vi "PDF Protokoll EPA1065_InterferenceVerification.vi"(8 "error in (no error)":errorcluster caption="Fehler (Eingang, kein Fehler)") -> (0 "error out":errorcluster caption="Fehler (Ausgang)")   [LabVIEW 2020, in "EPA 1065.lvlib" / "Interference verificaton 1065-375.lvlib"]
uses:
  Interference verificaton 1065-375.lvlib
  Visualisierungs Elemente/String - Ausgabefeld.ctl
  ResultTable.ctl
  Sprachverwaltung/FGV Aktion Tabelle zerlegen.ctl
  <vilib>/Utility/miscctls.llb/LVRowAndColumnTypeDef.ctl
  Aktion FGV Interference.ctl
  Seiten/FT-IR/FGV FT-IR Aktionen.ctl
  Aktion Index uebersetzten.ctl
  Seiten/System Einstellungen V2/Aktioen FGV System Konstanten.ctl
  <vilib>/Utility/miscctls.llb/LVPrintingMarginsTypeDef.ctl
  Allgemein/allgemeine Sub-VIs.lvlib
  Seiten/FT-IR/Span/Spanfaktor.lvlib
  Seiten/FT-IR/FT-IR.lvlib
  Sprachverwaltung/Sprachverwaltung.lvlib
  Seiten/System Einstellungen V2/System Einstellungen V2.lvlib
panel:
  out "[ppm]":sgl=1.0 caption="Limit:" min=0 format="%#.6g"
  out "[ppm]":sgl=120.0 caption="Interference:" min=0 format="%#.6g"
  out "LIN Ausgabetabelle":T1
  out "Komponente:":T2 caption="ppm"
  out "Tabelle 3":string[][](table)
  out "Tabelle":string[][](table)
  # "Interference Verification - EPA § 1065.375"
  # "Result"
  # "Analysis"
  # "Component:"
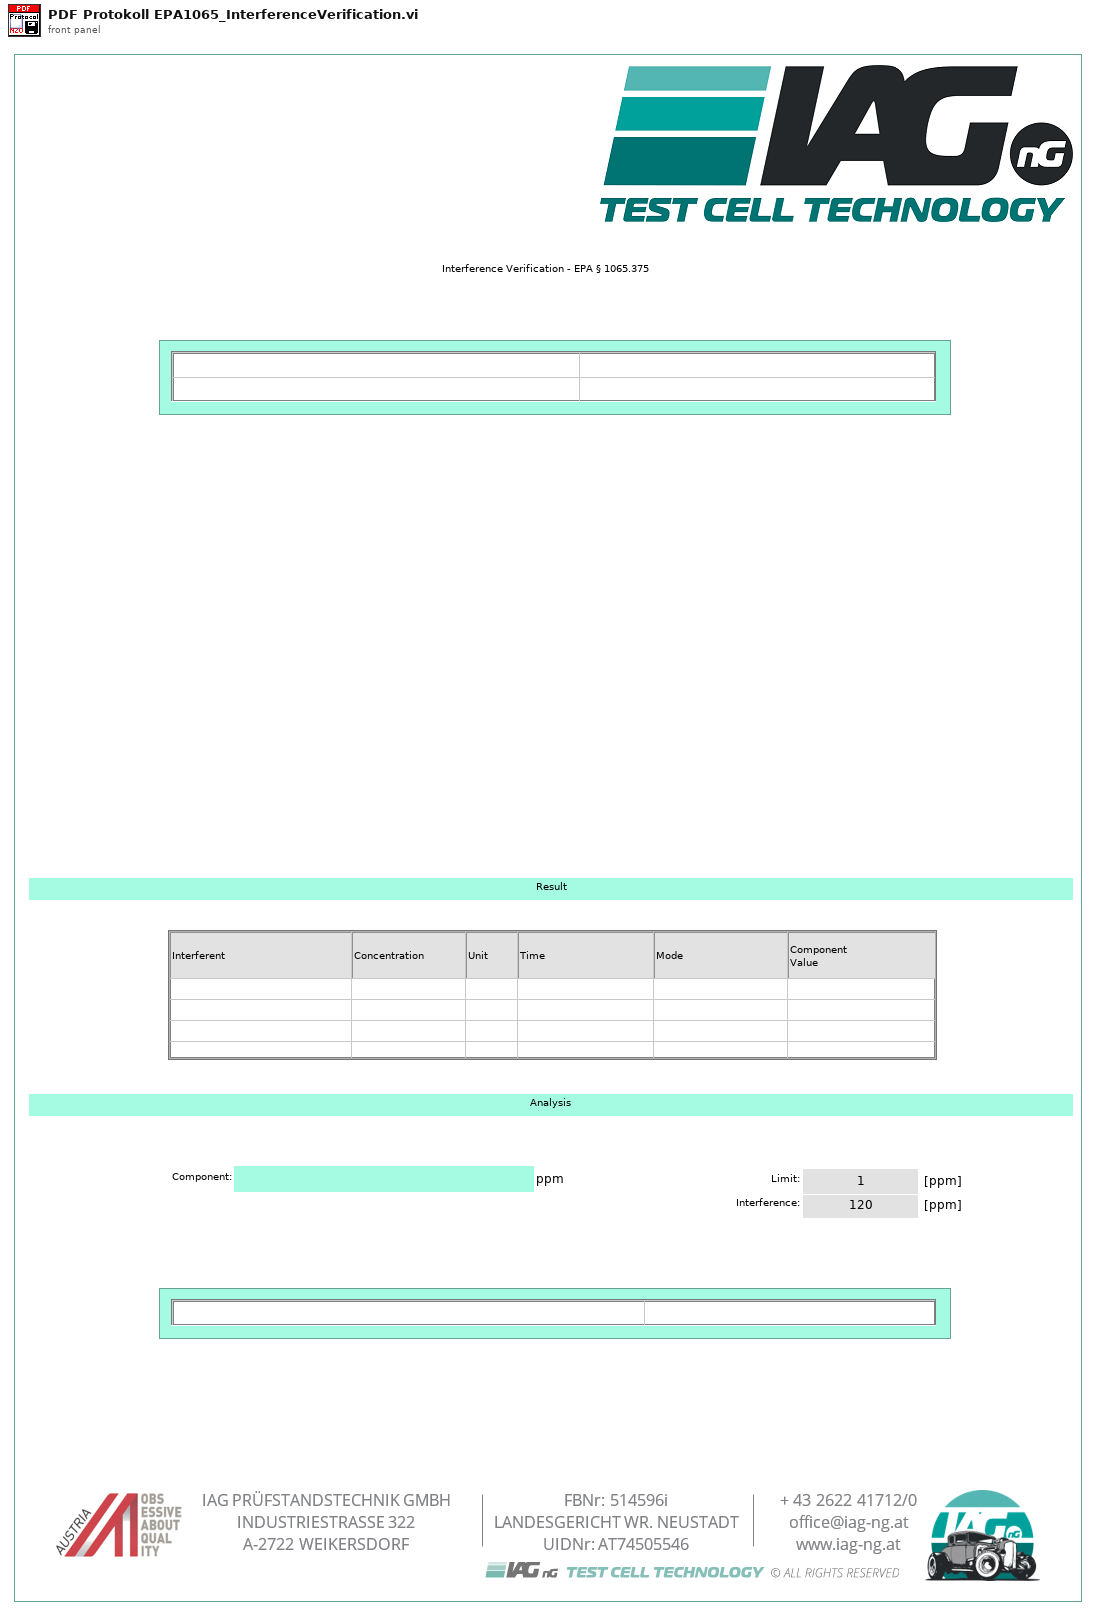
[diagram p1: front panel]
types:
  T1 = typedef "EPA 1065.lvlib/Interference verificaton 1065-375.lvlib/ResultTable.ctl" = string[][]
  T2 = typedef "String - Ausgabefeld.ctl" = string
  T3 = typedef "Sprachverwaltung.lvlib/FGV Aktion Tabelle zerlegen.ctl" = enum16{"laden", "vereinzeln", "speichern"}
  T4 = typedef "System Einstellungen V2.lvlib/Aktioen FGV System Konstanten.ctl" = enum16{"lesen", "laden", "speichern", "Sprache"}
  T5 = typedef "EPA 1065.lvlib/Interference verificaton 1065-375.lvlib/Aktion Index uebersetzten.ctl" = enum16{"lesen", "schreiben", "auswerten"}
  T6 = typedef "FT-IR.lvlib/FGV FT-IR Aktionen.ctl" = enum16{"lesen", "NOG setzen", "NOS setzen", "Initialisieren", "speichern", "ALLES setzen", "FT-IR Spektrum loggen", "Komm Stoppen", "Spektrum LogKonfig"}
  T7 = typedef "EPA 1065.lvlib/Interference verificaton 1065-375.lvlib/Aktion FGV Interference.ctl" = enum16{"Lesen", "TestKonfig", "TestSetting", "Einheiten", "Ergebnis", "Laden", "Tabelle", "Speichern", "löschen"}
  T8 = typedef "LVRowAndColumnTypeDef.ctl" = cluster{"Row":i32, "Column":i32}
  T9 = typedef "LVPrintingMarginsTypeDef.ctl" = cluster{"Top":sgl, "Left":sgl, "Bottom":sgl, "Right":sgl, "Measurement System":enum8{"Inches", "cm"}}
  T10 = enum32{"Portrait", "Landscape", "Rotated Portrait", "Rotated Landscape"}
  T11 = typedef "EPA 1065.lvlib/Interference verificaton 1065-375.lvlib/TestSetting.ctl" = cluster{"Bearbeiter:":string, "Pfad:":path, "Textname:":string, "Analysator":T12}
  T12 = typedef "System Einstellungen V2.lvlib/Analysatoren.ctl" = string
  T13 = typedef "EPA 1065.lvlib/Interference verificaton 1065-375.lvlib/TestKonfig.ctl" = cluster{"Komponente:":u16, "Modus":T14, "CG Aufschaltzeit:":dbl, "Interferent 1:":u16, "Interferent 2:":u16, "Interferent 3:":u16, "Gasflaschen Nr.:":string, "Gasflaschen Nr.: 2":string, "Gasflaschen Nr.: 3":string, "Inter 1 aktiv":bool, "Inter 2 aktiv":bool, "Inter 3 aktiv":bool, "Accuracy":string, "Accuracy 2":string, "Accuracy 3":string, "Konzentration 1:":dbl, "Konzentration 2:":dbl, "Konzentration 3:":dbl}
  T14 = typedef "EPA 1065.lvlib/Interference verificaton 1065-375.lvlib/Modus.ctl" = u16
  T15 = typedef "EPA 1065.lvlib/Interference verificaton 1065-375.lvlib/Komponenten.ctl" = cluster{"Komponente":T2, "Komponente Index":i32, "Komponente 2":T2, "Komponente Index 2":i32, "Komponente 3":T2, "Komponente Index 3":i32, "Interferent 1":T2, "Interferent Index":i32, "Interferent 2":T2, "Interferent 2 Index":i32, "Interferent 3":T2, "Interferent 3 Index":i32, "Interferent 4":T2, "Interferent 4 Index":i32}
  T16 = cluster{"Modell":string, "ProjektNummer":string, "Software Version":string, "Seriennummer":string}
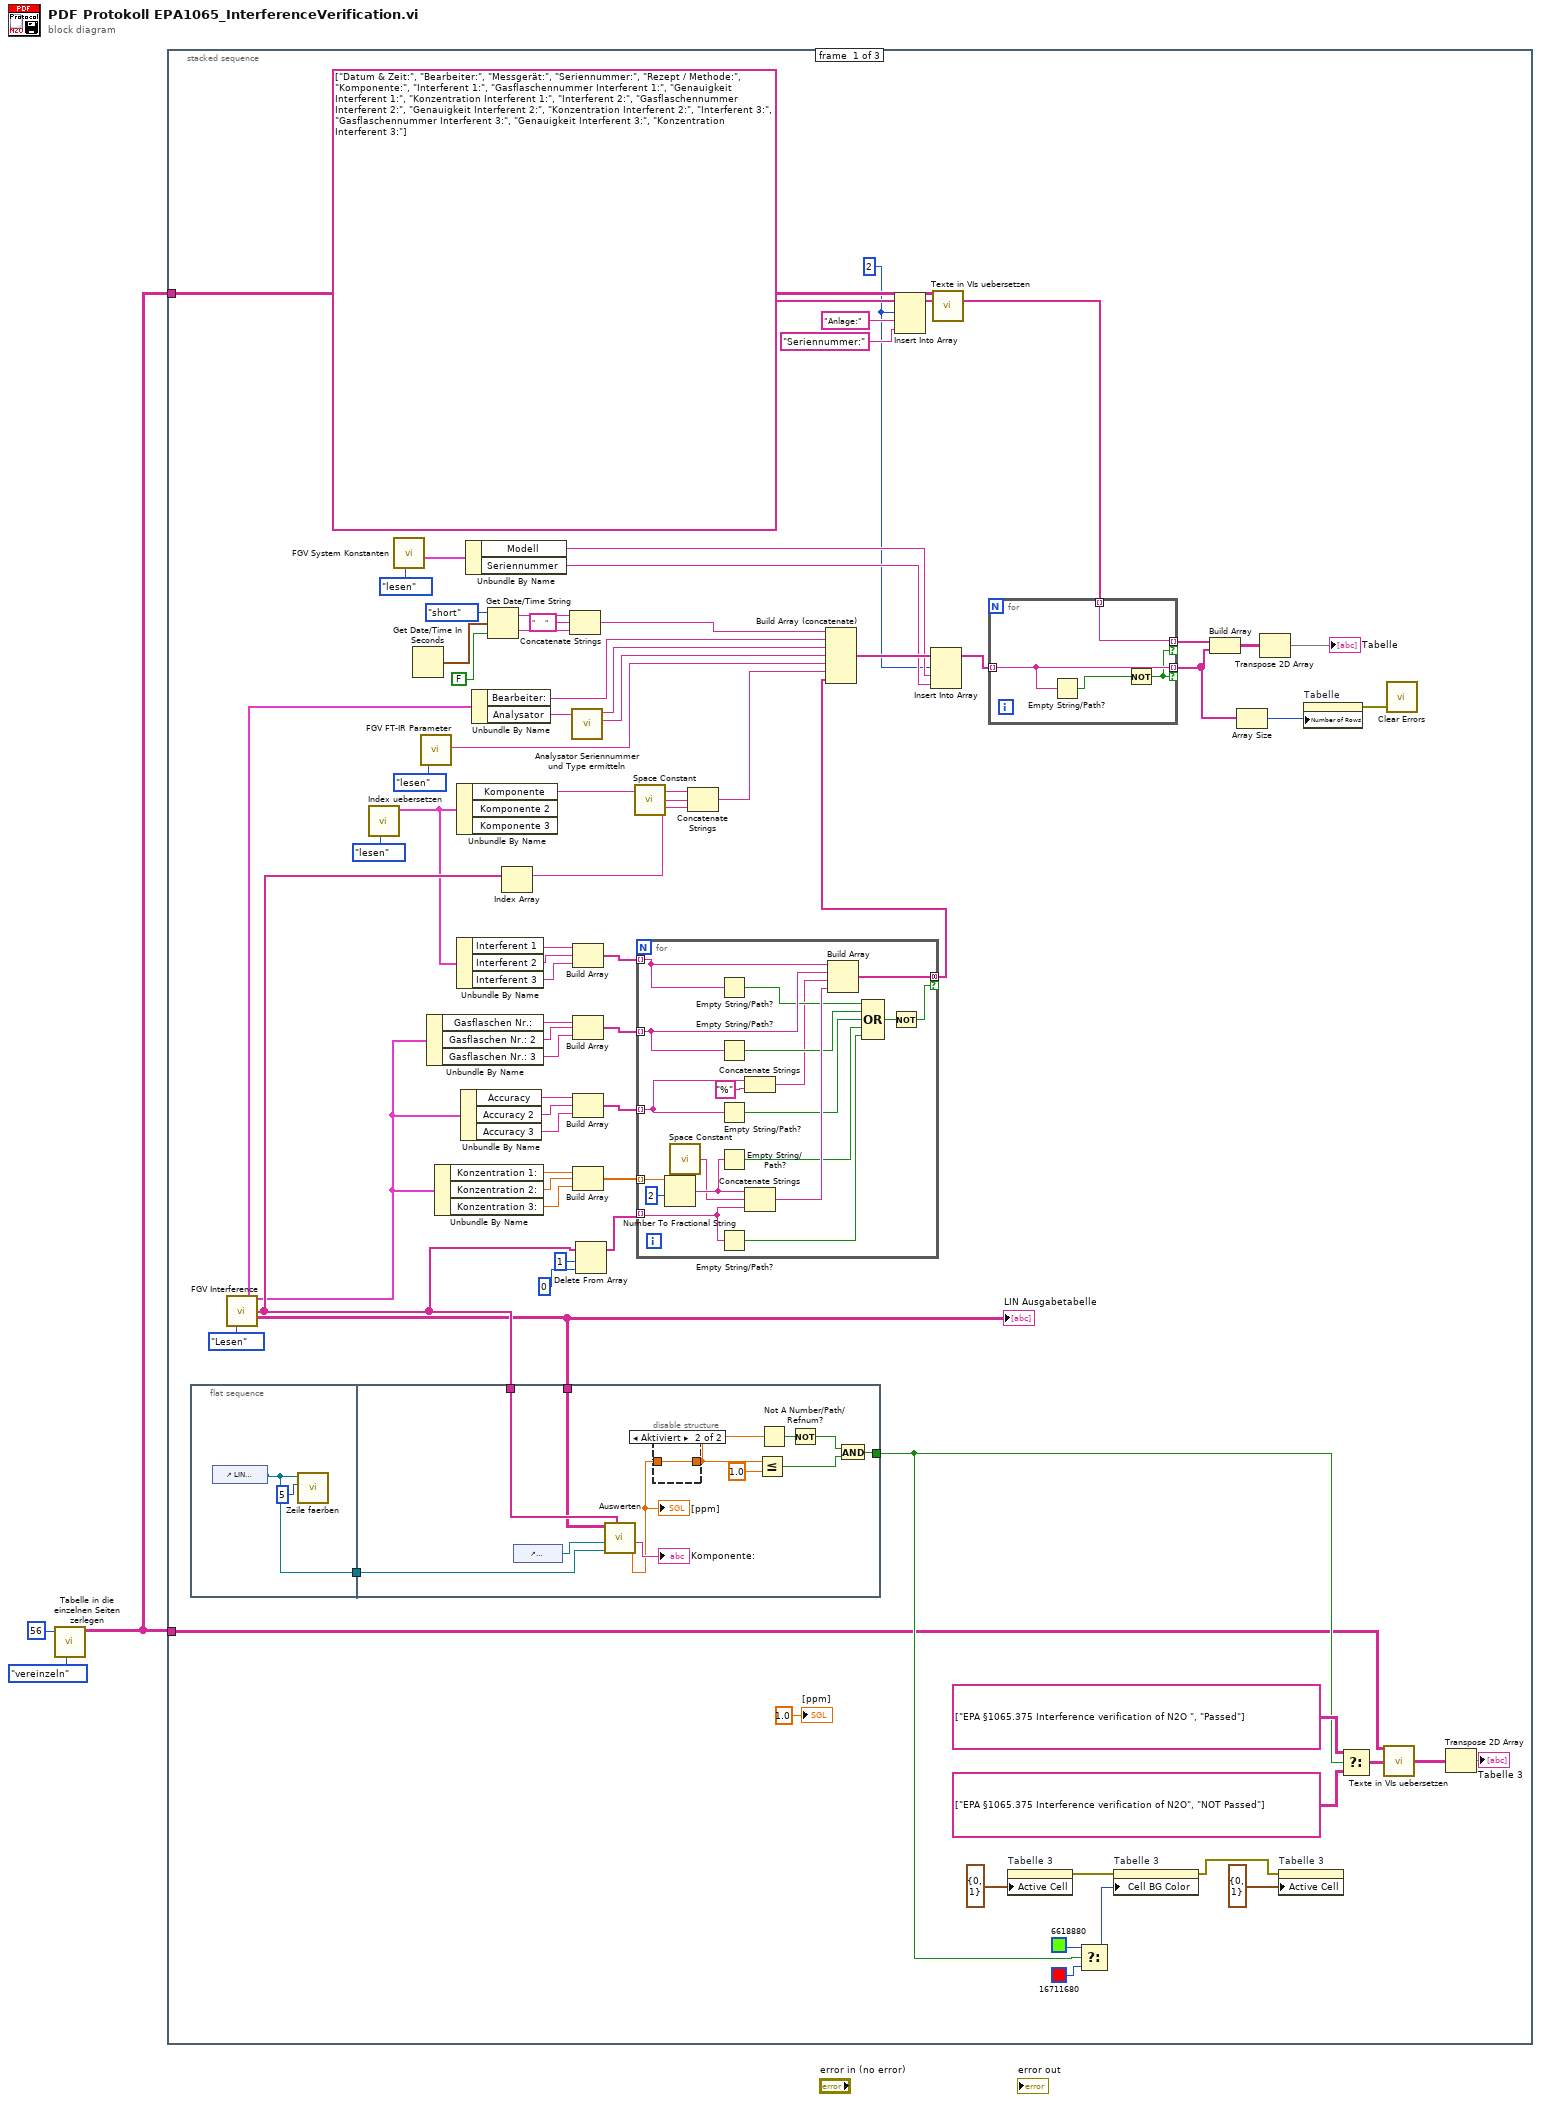
[diagram p0: block diagram]
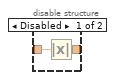
[diagram p2: hidden frame]
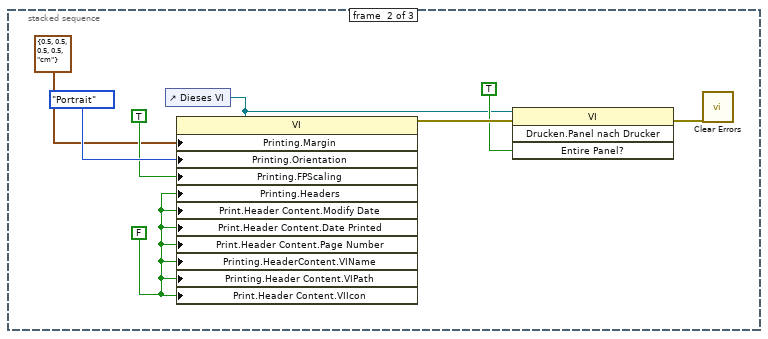
[diagram p3: hidden frame]
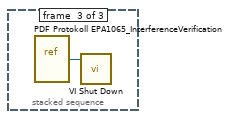
[diagram p4: hidden frame]
diagram:
  n1 = call "Tabelle in die einzelnen Seiten zerlegen.vi"("Aktion"=FGV_Aktion_Tabelle_zerlegen."vereinzeln", "Index (Seite)"=56) -> ("Sprachliste"=w1:string[][])  [unwired: 7 in, 2 out]
  n2 = stacked-sequence {
    tunnel: w1 -> [w24 _ _]
    tunnel: w1 -> [w22 _ _]
    frame #0 {
      w7 = 2 ("Index")
      n3 = flat-sequence {
        tunnel: [w106] -> w72
        tunnel: w72 -> [w119]
        tunnel: [w109] -> w71
        tunnel: w50 -> [w115]
        tunnel: w27 -> [w114]
        frame #0 {
          n4 = control-ref of="LIN Ausgabetabelle"() -> (w106:refnum<vi>)
          n5 = call "Zeile faerben.vi"("Anzahl"=5, "Table (Eingang)"=w106) -> ()  [unwired: 9 in, 1 out]
        }
        frame #1 {
          n6 = control-ref of="Komponente:"() -> (w117:refnum<vi>)
          n7 = call "Auswerten.vi"("Êinheiten"=w115, "LIN Ausgabetabelle"=w119, "Komponente:"=w117, "Tabelle"=w114) -> ("Konzentration Komponente"=w108:dbl, "Komponente:"=→"Komponente:":T2)  [unwired: 4 in, 2 out]
          "[ppm]" <- w108
          n8 = disable-structure shown="Aktiviert" {
            disable-tunnel: [w121 w122] -> w113
            disable-tunnel: w108 -> [w120 w122]
            frame Disabled {
              n9 = Absolute Value(x=w120) -> (abs(x)=w121:dbl)
            }
            frame Enabled {
            }
          }
          n10 = Less Or Equal?(x=w113, y=1.0) -> (x <= y?=w111:bool)
          n11 = Not A Number/Path/Refnum?(number/path/refnum=w113) -> (NaN/Path/Refnum?=w112:bool)
          n12 = Not(x=w112) -> (.not. x?=w110:bool)
          n13 = And(x=w110, y=w111) -> (x .and. y?=w109:bool)
        }
      }
      n14 = call "FGV Interference.vi"("Aktion FGV Interference"=Aktion_FGV_Interference."Lesen") -> ("TestSetting"=w69:T11, "TestKonfig 2"=w32:T13, "Êinheiten"=w50:string[], "Tabelle"=w27:T2[][])  [unwired: 9 in, 2 out]
      "LIN Ausgabetabelle" <- w27
      n15 = call "Index uebersetzen.vi"("Aktion"=Aktion_Index_uebersetzten."lesen") -> ("Komponenten"=w45:T15)  [unwired: 9 in, 1 out]
      n16 = call "FGV System Konstanten.vi"("Aktionen"=Aktioen_FGV_System_Konstanten."lesen") -> ("Cluster out"=w16:T16)  [unwired: 6 in, 4 out]
      n17 = Get Date/Time In Seconds() -> (seconds since 1Jan1904=w68:timestamp)
      n18 = call "FGV FT-IR Parameter.vi"("Aktion"=FGV_FT-IR_Aktionen."lesen") -> ("Current Recipe"=w57:string)  [unwired: 11 in, 7 out]
      n19 = Unbundle By Name(w32) -> ("Gasflaschen Nr.:"=w44:string, "Gasflaschen Nr.: 2"=w43:string, "Gasflaschen Nr.: 3"=w42:string)
      n20 = Unbundle By Name(w32) -> ("Konzentration 1:"=w41:dbl, "Konzentration 2:"=w40:dbl, "Konzentration 3:"=w39:dbl)
      n21 = Unbundle By Name(w45) -> ("Komponente"=w20:T2)  [unwired: 2 out]
      n22 = Unbundle By Name(w45) -> ("Interferent 1"=w48:T2, "Interferent 2"=w47:T2, "Interferent 3"=w46:T2)
      n23 = Unbundle By Name(w32) -> ("Accuracy"=w31:string, "Accuracy 2"=w30:string, "Accuracy 3"=w29:string)
      n24 = Unbundle By Name(w16) -> ("Modell"=w9:string, "Seriennummer"=w8:string)
      n25 = Unbundle By Name(w69) -> ("Bearbeiter:"=w59:string, "Analysator"=w6:T12)
      n26 = Get Date/Time String(date format (0)=enum16{"short", "long", "abbreviated"}."short" ("Datumsformat (0)"), seconds (now)=w68, want seconds? (F)=FALSE ("Angabe von Sekunden? (F)")) -> (date string=w67:string, time string=w66:string)
      n27 = Index Array(array=w50) -> (element=w19:string)  [unwired: 1 in]
      n28 = Concatenate Strings(w67, "     " ("String"), w66) -> (w60:string)
      n29 = call "Analysator Seriennummer und Type ermitteln.vi"("Analysator"=w6) -> ("Type"=w4:string, "Name für Protokoll"=w5:string)  [unwired: 8 in, 1 out]
      n30 = Build Array(w48, w47, w46) -> (w38:T2[])
      n31 = Build Array(w44, w43, w42) -> (w37:string[])
      n32 = Build Array(w31, w30, w29) -> (w28:string[])
      n33 = Build Array(w41, w40, w39) -> (w36:dbl[])
      n34 = Delete From Array(array=w50, length=1 ("Länge"), index=0 ("Index")) -> (array with subset deleted=w34:string[])  [unwired: 1 out]
      n35 = call <vilib>:"Space Constant.vi"() -> ("String"=w21:string)
      n36 = for {
        tunnel: w38 -> [w98] mode=indexing
        tunnel: w37 -> [w97] mode=indexing
        tunnel: w36 -> [w101] mode=indexing
        tunnel: w34 -> [w100] mode=indexing
        tunnel: [w95] -> w33 mode=concatenating if=w83
        tunnel: w28 -> [w84] mode=indexing
        n37 = Number To Fractional String(number=w101, precision (6)=i16 2 ("Genauigkeit (6)")) -> (F-format string=w99:string)  [unwired: 2 in]
        n38 = call <vilib>:"Space Constant.vi"() -> ("String"=w89:string)
        n39 = Empty String/Path?(string/path=w98) -> (empty?=w94:bool)
        n40 = Empty String/Path?(string/path=w97) -> (empty?=w93:bool)
        n41 = Empty String/Path?(string/path=w84) -> (empty?=w85:bool)
        n42 = Empty String/Path?(string/path=w99) -> (empty?=w90:bool)
        n43 = Empty String/Path?(string/path=w100) -> (empty?=w92:bool)
        n44 = Concatenate Strings(w84, "%" ("String")) -> (w87:string)
        n45 = Concatenate Strings(w99, w89, w100) -> (w96:string)
        n46 = Build Array(w98, w97, w87, w96) -> (w95:T2[])
        n47 = Compound Arithmetic op=OR ("Mehrfacharithmetik")(w94, w93, w85, w90, w92) -> (w91:bool)
        n48 = Not(x=w91) -> (.not. x?=w83:bool)
      }
      n49 = Concatenate Strings(w20, w21, w19) -> (w58:string)
      n50 = Build Array (concatenate)(w60, w59, w5, w4, w57, w58, w33) -> (w11:T2[])
      n51 = Insert Into Array(array=string[] ["Datum & Zeit:", "Bearbeiter:", "Messgerät:", "Seriennummer:", "Rezept / Methode:", "Komponente:", "Interferent 1:", "Gasflaschennummer Interferent 1:", "Genauigkeit Interferent 1:", "Konzentration Interferent 1:", "Interferent 2:", "Gasflaschennummer Interferent 2:", "Genauigkeit Interferent 2:", "Konzentration Interferent 2:", "Interferent 3:", "Gasflaschennummer Interferent 3:", "Genauigkeit Interferent 3:", "Konzentration Interferent 3:"], index=w7, new element #1="Anlage:" ("Neues Element/Teil-Array"), new element #2="Seriennummer:" ("Neues Element/Teil-Array")) -> (w12:string[])
      n52 = Insert Into Array(array=w11, index=w7, new element #1=w9, new element #2=w8) -> (w10:T2[])
      n53 = call "Texte in VIs uebersetzen.vi"("Sprachliste"=w22, "String-Array zum Übersetzen"=w12) -> ("String-Array zum Übersetzen"=w23:string[])  [unwired: 9 in, 4 out]
      n54 = for {
        tunnel: w10 -> [w105] mode=indexing
        tunnel: [w105] -> w53 mode=indexing if=w102
        tunnel: [w103] -> w56 mode=indexing if=w102
        tunnel: w23 -> [w103] mode=indexing
        n55 = Empty String/Path?(string/path=w105) -> (empty?=w104:bool)
        n56 = Not(x=w104) -> (.not. x?=w102:bool)
      }
      n57 = property on="Tabelle 3" class="Tbl (strikt)"("Active Cell"=T8 {"Row"=0, "Column"=1} ("Aktive Zelle:Aktive Zelle")) -> (error out=w78:errorcluster)  [unwired: 2 in, 1 out]
      n58 = Select(t=u32 6618880, s=w71, f=u32 16711680) -> (s? t:f=w79:u32)
      n59 = property on="Tabelle 3" class="Tbl (strikt)"(error in=w78, "Cell BG Color"=w79) -> (error out=w73:errorcluster)  [unwired: 1 in, 1 out]
      n60 = Build Array(w56, w53) -> (w55:T2[][])
      n61 = Array Size(array=w53) -> (size(s)=w52:i32)
      n62 = Transpose 2D Array(2D array=w55) -> (transposed array=→"Tabelle":T2[][])
      n63 = property on="Tabelle 3" class="Tbl (strikt)"(error in=w73, "Active Cell"=T8 {"Row"=0, "Column"=1} ("Aktive Zelle:Aktive Zelle")) -> ()  [unwired: 1 in, 2 out]
      n64 = property on="Tabelle" class="Tbl (strikt)"("Number of Rows"=w52) -> (error out=w51:errorcluster)  [unwired: 2 in, 1 out]
      n65 = Select(t=string[][] [["EPA §1065.375 Interference verification of N2O "], ["Passed"]] ("Tabelle 3"), s=w71, f=string[][] [["EPA §1065.375 Interference verification of N2O"], ["NOT Passed"]] ("Tabelle 3")) -> (s? t:f=w26:string[][])
      n66 = call "Texte in VIs uebersetzen.vi"("Sprachliste"=w24, "2D String-Array zum Übersetzen"=w26) -> ("2D String-Array zum Übersetzen"=w25:string[][])  [unwired: 9 in, 4 out]
      n67 = call <vilib>:"Clear Errors.vi"("error in (no error)"=w51) -> ()  [unwired: 5 in, 2 out]
      n68 = Transpose 2D Array(2D array=w25) -> (transposed array=→"Tabelle 3":string[][])
      "[ppm]" <- sgl 1.0 ("[ppm]")
    }
    frame #1 {
      w126 = FALSE ("Drucken:Kopfzeilen?")
      n69 = control-ref of="Dieses VI"() -> (w123:refnum<vi>)
      n70 = property class="VI"(reference=w123, "Printing.Margin"=T9 {"Top"=0.5, "Left"=0.5, "Bottom"=0.5, "Right"=0.5, "Measurement System"=enum."cm"} ("Drucken:Ränder"), "Printing.Orientation"=T10."Portrait" ("Drucken:Seitenausrichtung"), "Printing.FPScaling"=TRUE ("Drucken:Frontpanel-Skalierung?"), "Printing.Headers"=w126, "Print.Header Content.Modify Date"=w126, "Print.Header Content.Date Printed"=w126, "Print.Header Content.Page Number"=w126, "Printing.HeaderContent.VIName"=w126, "Printing.Header Content.VIPath"=w126, "Print.Header Content.VIIcon"=w126) -> (error out=w130:errorcluster)  [unwired: 1 in, 1 out]
      n71 = invoke class="VI" method="Drucken.Panel nach Drucker"(reference=w123, error in=w130, "Entire Panel?"=TRUE ("Abschnittskopfzeilen?")) -> (error out=w124:errorcluster)  [unwired: 1 in, 3 out]
      n72 = call <vilib>:"Clear Errors.vi"("error in (no error)"=w124) -> ()  [unwired: 5 in, 2 out]
    }
    frame #2 {
      n73 = vi-ref "PDF Protokoll EPA1065_InterferenceVerification.vi"() -> (w131:refnum<vi>)
      n74 = call "VI Shut Down.vi"("VI Referenz"=w131) -> ()  [unwired: 11 in]
    }
  }
